vi "Calculate Velocity Setpoints.vi"(4 "Commands":cluster{"Time (s)":dbl, T1, bool}[](array[cluster]), 5 "Reset Accumulator":bool, 6 "Booleans":T3, 8 "Iterations":dbl, 9 "IMU":dbl, 10 "Angles":dbl[](array[numeric]), 11 "Velocity":dbl[](array[numeric])) -> (0 "Finished":bool, 1 "Left Velocity":dbl, 2 "Right Velocity":dbl)   [LabVIEW 2019]
uses:
  Bordeaux/bordeaux-pathinator/Bordeaux/Command Stuff/Single Cmd Info.ctl
  <vilib>/picture/picture.llb/imagedata.ctl
  <vilib>/addons/control/pid/pid.llb/PID (DBL).vi
  <vilib>/addons/control/pid/NI_PID_pid.lvlib
panel:
  out "IMU":cluster{"Combined Angle":dbl, "IMU":dbl}(graph)
  in  "Turn Radius":dbl=1.0
  in  "PID gains":T4={"proportional gain (Kc)"=0.08, "integral time (Ti, min)"=0.0, "derivative time (Td, min)"=0.0} {"derivative time (Td, min)" format="%.5f"; "integral time (Ti, min)" format="%.6f"; "proportional gain (Kc)" format="%.6f"}
  in  "IMU":bool=TRUE
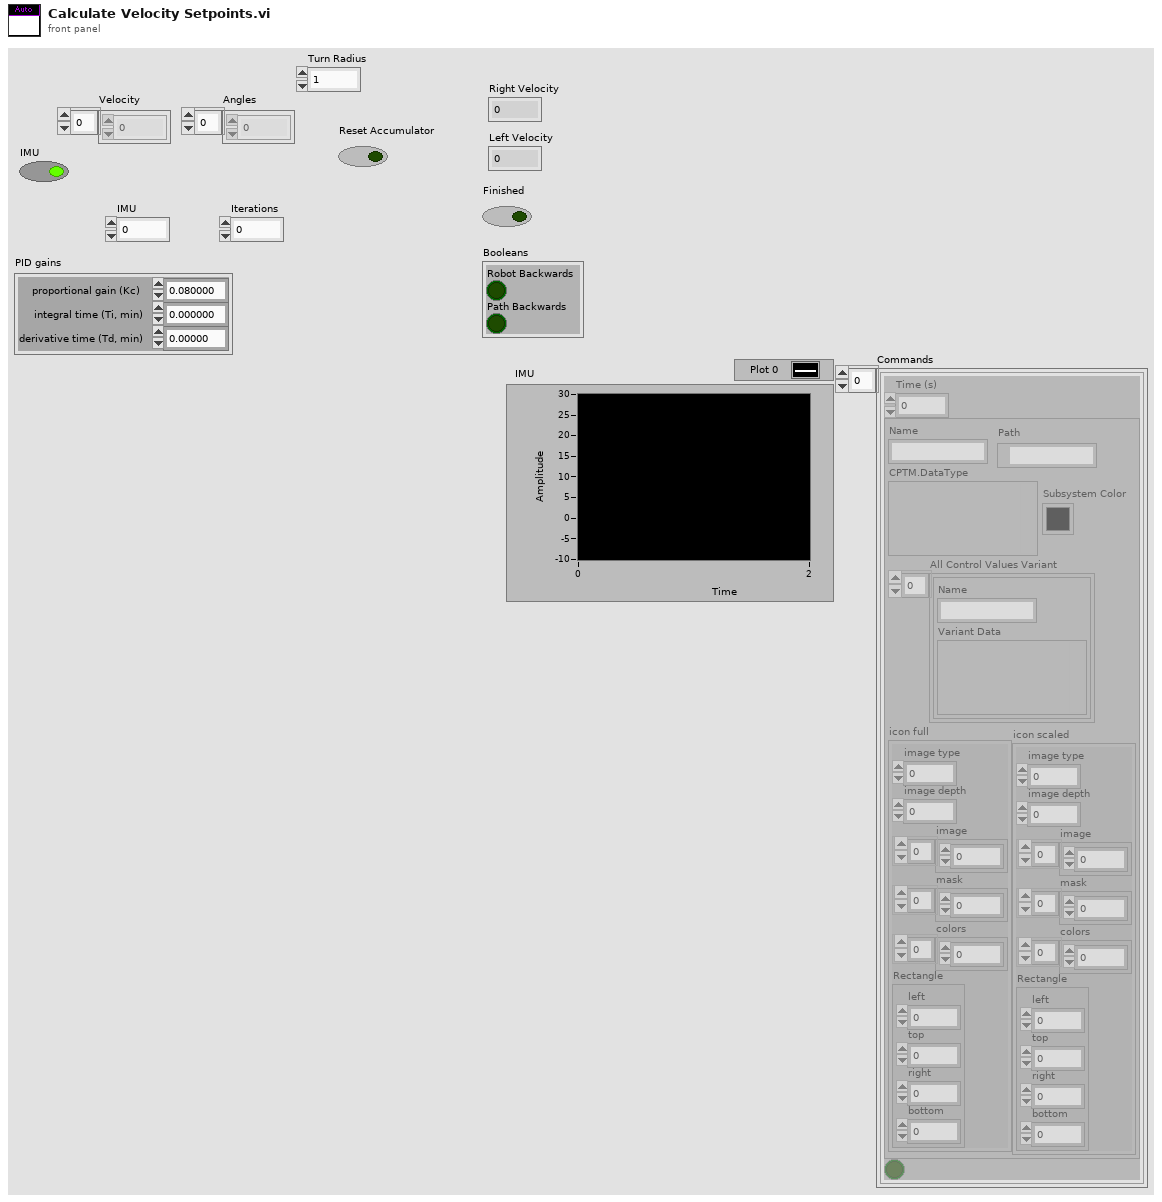
[diagram p1: front panel]
types:
  T1 = typedef "Single Cmd Info.ctl" = cluster{"Name":string, "CPTM.DataType":variant, "All Control Values Variant":cluster{"Name":string, "Variant Data":variant}[], "icon full":T2, "icon scaled":T2, "Path":path, "Subsystem Color":u32}
  T2 = typedef "imagedata.ctl" = cluster{"image type":i32, "image depth":i32, "image":u8[], "mask":u8[], "colors":u32[], "Rectangle":cluster{"left":i16, "top":i16, "right":i16, "bottom":i16}}
  T3 = cluster{"Robot Backwards":bool, "Path Backwards":bool}
  T4 = cluster{"proportional gain (Kc)":dbl, "integral time (Ti, min)":dbl, "derivative time (Td, min)":dbl}
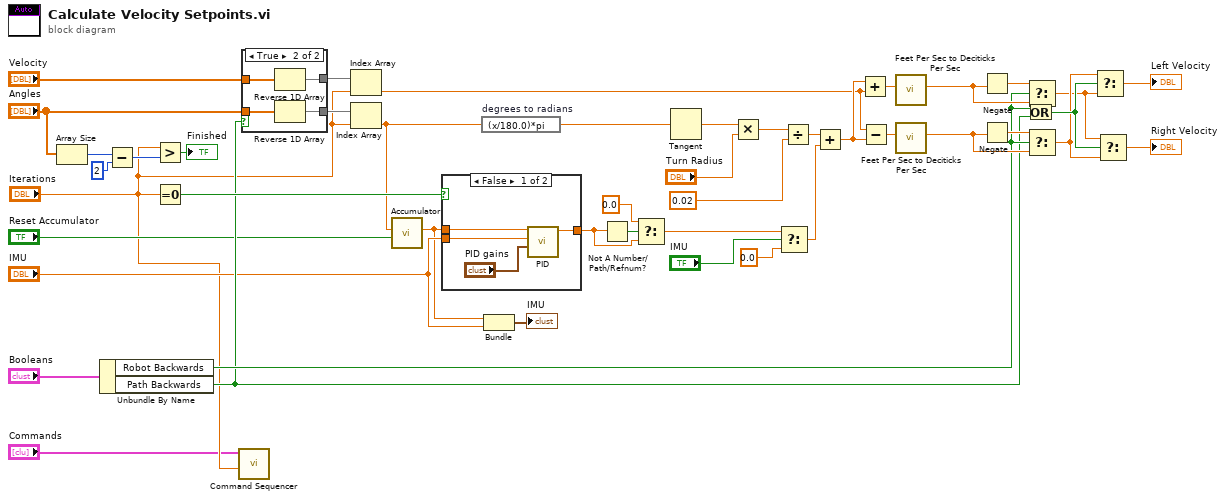
[diagram p0: block diagram]
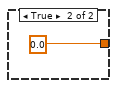
[diagram p3: hidden frame]
diagram:
  n1 = Array Size(array="Angles") -> (size(s)=w39:i32)
  n2 = Unbundle By Name("Booleans") -> ("Robot Backwards"=w28:bool, "Path Backwards"=w27:bool)
  n3 = Subtract(x=w39, y=2) -> (x-y=w3:i32)
  n4 = Greater?(x="Iterations", y=w3) -> (0:→"Finished":bool)
  n5 = Equal To 0?(x="Iterations") -> (x = 0?=w42:bool)
  n6 = call "Command Sequencer.vi"("Iterations"="Iterations", "Commands"="Commands") -> ()  [unwired: 9 in, 1 out]
  n7 = case shown="True" w27 {
    tunnel: "Velocity" -> [w47 w51]
    tunnel: "Angles" -> [w46 w50]
    tunnel: [w46 w49] -> w30
    tunnel: [w47 w48] -> w29
    frame False {
    }
    frame True {
      n8 = Reverse 1D Array(array=w51) -> (reversed array=w48:dbl[])
      n9 = Reverse 1D Array(array=w50) -> (reversed array=w49:dbl[])
    }
  }
  n10 = Index Array(array=w29, index="Iterations") -> (element=w15:dbl)
  n11 = Index Array(array=w30, index="Iterations") -> (element=w21:dbl)
  n12 = call "Accumulator.vi"("Reset Accumulator"="Reset Accumulator", "Delta Angle"=w21) -> ("Combined Angle"=w16:dbl)  [unwired: 9 in]
  n13 = case shown="False" w42 {
    tunnel: [w55 0.0 ("output")] -> w11
    tunnel: "IMU" -> [w54 _]
    tunnel: w16 -> [w53 _]
    frame False {
      n14 = call-poly <vilib>:"PID.vi"("PID gains"="PID gains", "process variable"=w54, "setpoint"=w53) -> ("output"=w55:dbl)  [unwired: 7 in, 1 out]
    }
    frame True {
    }
  }
  n15 = expression code="(x/180.0)*pi" "degrees to radians"(w21) -> (w9:dbl)
  n16 = Bundle("Combined Angle"=w16, "IMU"="IMU") -> (→"IMU":cluster{"Combined Angle":dbl, "IMU":dbl})  [unwired: 1 in]
  n17 = Not A Number/Path/Refnum?(number/path/refnum=w11) -> (NaN/Path/Refnum?=w14:bool)
  n18 = Select(t=0.0, s=w14, f=w11) -> (s? t:f=w13:dbl)
  n19 = Tangent(1:w9) -> (0:w26:dbl)
  n20 = Multiply(x=w26, y="Turn Radius") -> (x*y=w23:dbl)
  n21 = Select(t=w13, s="IMU", f=0.0 ("x")) -> (s? t:f=w24:dbl)
  n22 = Divide(x=w23, y=0.02) -> (x/y=w22:dbl)
  n23 = Add(x=w22, y=w24) -> (x+y=w45:dbl)
  n24 = Add(x=w45, y=w15) -> (x+y=w40:dbl)
  n25 = Subtract(x=w15, y=w45) -> (x-y=w41:dbl)
  n26 = call "Feet Per Sec to Deciticks Per Sec.vi"("Ft/Sec"=w40) -> ("DeciTick/Sec"=w35:dbl)  [unwired: 10 in]
  n27 = call "Feet Per Sec to Deciticks Per Sec.vi"("Ft/Sec"=w41) -> ("DeciTick/Sec"=w33:dbl)  [unwired: 10 in]
  n28 = Negate(x=w35) -> (-x=w36:dbl)
  n29 = Negate(x=w33) -> (-x=w34:dbl)
  n30 = Or(x=w28, y=w27) -> (x .or. y?=w8:bool)
  n31 = Select(t=w36, s=w28, f=w35) -> (s? t:f=w6:dbl)
  n32 = Select(t=w34, s=w28, f=w33) -> (s? t:f=w7:dbl)
  n33 = Select(t=w7, s=w8, f=w6) -> (s? t:f=→"Left Velocity":dbl)
  n34 = Select(t=w6, s=w8, f=w7) -> (s? t:f=→"Right Velocity":dbl)
